vi "InstrumentSelection.vi"(8 "error in (no error)":errorcluster, 9 "Verify GPIB address":bool, 10 "Instrument type":enum16{"Supply", "LCR", "Multimeter"}(ring), 11 "Instrument name IN":string(combo)) -> (0 "error out":errorcluster, 1 "Instrument name OUT":string, 2 "LCR":refnum<class "LCRControl.lvclass">, 3 "Supply":refnum<class "SupplyControl.lvclass">, 5 "Multimeter":refnum<class "MultimeterControl.lvclass">)   [LabVIEW 2018, in "InstrControl.lvclass"]
uses:
  InstrControl.lvclass
  SupplyControl/SupplyControl.lvclass
  C:/ProbeTestSoftware2019/itk-strip-sensor-qc/InstrControl/InstrControl.lvclass
  LCRControl/LCRControl.lvclass
  MultimeterControl/MultimeterControl.lvclass
  SupplyControl/Keithley 2410/KE2410.lvclass
  C:/ProbeTestSoftware2019/itk-strip-sensor-qc/InstrControl/SupplyControl/SupplyControl.lvclass
  SupplyControl/Keithley 6517/KE6517.lvclass
  SupplyControl/Keithley 487/KE487.lvclass
  SupplyControl/Keithley 2657A/KE2657A.lvclass
  SupplyControl/Keithley 236 & 237/KE236.lvclass
  LCRControl/WK6440B/WK6440B.lvclass
  C:/ProbeTestSoftware2019/itk-strip-sensor-qc/InstrControl/LCRControl/LCRControl.lvclass
  LCRControl/WK6425/WK6425.lvclass
  MultimeterControl/Keithley 2000/KE2000.lvclass
  C:/ProbeTestSoftware2019/itk-strip-sensor-qc/InstrControl/MultimeterControl/MultimeterControl.lvclass
  InstrumentSetup.vi
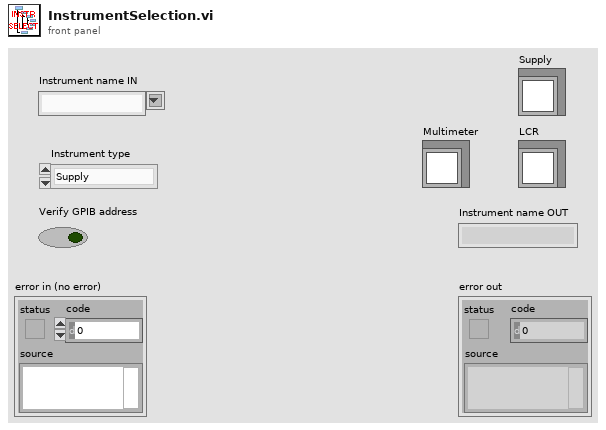
[diagram p1: front panel]
types:
  T1 = cluster{"KE 2410":cluster{"Instrument name":string, "GPIB address":string, "Instrument type":u16}, "KE 6517":cluster{"Instrument name":string, "GPIB address":string, "Instrument type":u16}, "KE 487":cluster{"Instrument name":string, "GPIB address":string, "Instrument type":u16}, "KE 2657A":cluster{"Instrument name":string, "GPIB address":string, "Instrument type":u16}, "KE 236":cluster{"Instrument name":string, "GPIB address":string, "Instrument type":u16}, "WK 6440B":cluster{"Instrument name":string, "GPIB address":string, "Instrument type":u16}, "WK 6425":cluster{"Instrument name":string, "GPIB address":string, "Instrument type":u16}, "Pickering Matrix":cluster{"Instrument name":string, "GPIB address":string, "Instrument type":u16}, "KE 2000":cluster{"Instrument name":string, "GPIB address":string, "Instrument type":u16}}
  T2 = cluster{"current \ncompliance level":dbl, "compliance/\nmeasurement range (auto:0)":u16}
  T3 = cluster{"RC Configuration":u16, "AC amplitude [V]":dbl, "AC frequency [Hz]":i32}
  T4 = cluster{"Range":u16, "Range Value":dbl, "Function":u16}
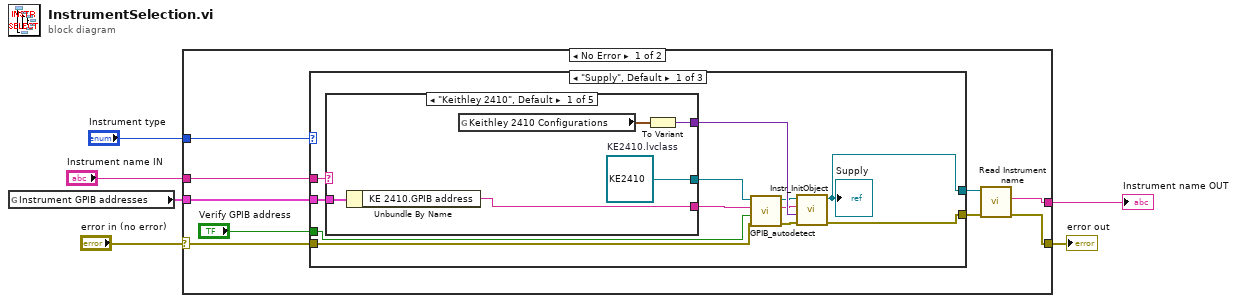
[diagram p0: block diagram]
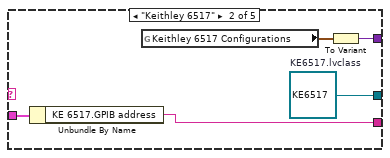
[diagram p2: hidden frame]
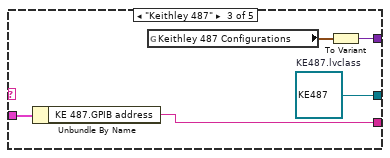
[diagram p3: hidden frame]
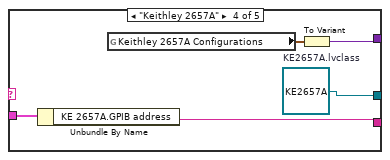
[diagram p4: hidden frame]
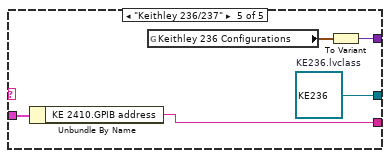
[diagram p5: hidden frame]
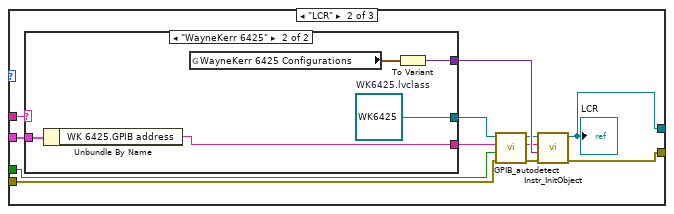
[diagram p6: hidden frame]
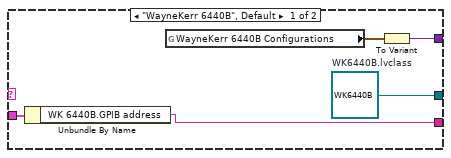
[diagram p7: hidden frame]
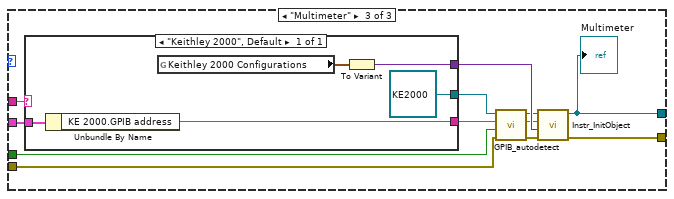
[diagram p8: hidden frame]
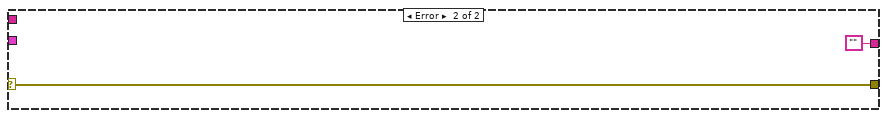
[diagram p9: hidden frame]
diagram:
  n1 = global read "InstrumentSetup.vi" "Instrument GPIB addresses"() -> (w1:T1)
  n2 = case shown="No Error" "error in (no error)" {
    selector: "error in (no error)" -> [w13 w93]
    tunnel: [w14 w93] -> w5
    tunnel: [w15 ""] -> w4
    tunnel: "Instrument type" -> [w10 _]
    tunnel: "Instrument name IN" -> [w9 _]
    tunnel: w1 -> [w8 _]
    frame No Error {
      n3 = case shown="\"Supply\", Default" w10 {
        tunnel: w9 -> [w27 w64 w86]
        tunnel: [w26 w62 w84] -> w12
        tunnel: w13 -> [w18 w59 w76]
        tunnel: [w25 w63 w85] -> w11
        tunnel: w8 -> [w24 w61 w83]
        tunnel: "Verify GPIB address" -> [w17 w53 w81]
        frame "Supply", Default {
          n4 = case shown="\"Keithley 2410\", Default" w27 {
            tunnel: [w32 w37 w42 w43 w52] -> w20
            tunnel: w24 -> [w31 w36 w41 w45 w51]
            tunnel: [w30 w35 w40 w44 w50] -> w22
            tunnel: [w28 w33 w39 w46 w48] -> w23
            frame "Keithley 2410", Default {
              w32 = refnum<class "KE2410.lvclass"> refnum  # KE2410.lvclass
              n5 = Unbundle By Name(w31) -> ("KE 2410.GPIB address"=w30:string)
              n6 = global read "InstrumentSetup.vi" "Keithley 2410 Configurations"() -> (w29:cluster{"Current Limit":sgl})
              n7 = To Variant(anything=w29) -> (Variant=w28:variant)
            }
            frame "Keithley 6517" {
              w37 = refnum<class "KE6517.lvclass"> refnum  # KE6517.lvclass
              n8 = Unbundle By Name(w36) -> ("KE 6517.GPIB address"=w35:string)
              n9 = global read "InstrumentSetup.vi" "Keithley 6517 Configurations"() -> (w34:cluster{"Current Limit":u16})
              n10 = To Variant(anything=w34) -> (Variant=w33:variant)
            }
            frame "Keithley 487" {
              w42 = refnum<class "KE487.lvclass"> refnum  # KE487.lvclass
              n11 = Unbundle By Name(w41) -> ("KE 487.GPIB address"=w40:string)
              n12 = global read "InstrumentSetup.vi" "Keithley 487 Configurations"() -> (w38:cluster{"Compliance":u16, "Range:":u16})
              n13 = To Variant(anything=w38) -> (Variant=w39:variant)
            }
            frame "Keithley 2657A" {
              w43 = refnum<class "KE2657A.lvclass"> refnum  # KE2657A.lvclass
              n14 = Unbundle By Name(w45) -> ("KE 2657A.GPIB address"=w44:string)
              n15 = global read "InstrumentSetup.vi" "Keithley 2657A Configurations"() -> (w47:cluster{"Current Limit":sgl})
              n16 = To Variant(anything=w47) -> (Variant=w46:variant)
            }
            frame "Keithley 236/237" {
              w52 = refnum<class "KE236.lvclass"> refnum  # KE236.lvclass
              n17 = Unbundle By Name(w51) -> ("KE 2410.GPIB address"=w50:string)
              n18 = global read "InstrumentSetup.vi" "Keithley 236 Configurations"() -> (w49:T2)
              n19 = To Variant(anything=w49) -> (Variant=w48:variant)
            }
          }
          n20 = call-dynamic "GPIB_autodetect.vi"("error in (no error)"=w18, "Verify GPIB address"=w17, "Instrument GPIB address in"=w22, "InstrControl in"=w20) -> ("error out"=w16:errorcluster, "Instrument GPIB address"=w21:string, "InstrControl out"=w19:refnum<class "SupplyControl.lvclass">)  [unwired: 5 in]
          n21 = call-dynamic "Instr_InitObject.vi"("error in (no error)"=w16, "Instrument Configuration"=w23, "GPIB address"=w21, "SupplyControl in"=w19) -> ("error out"=w25:errorcluster, "SupplyControl out"=w26:refnum<class "SupplyControl.lvclass">)  [unwired: 6 in]
          "Supply" <- w26
        }
        frame "LCR" {
          n22 = case shown="\"WayneKerr 6425\"" w64 {
            tunnel: [w69 w74] -> w55
            tunnel: w61 -> [w68 w73]
            tunnel: [w67 w72] -> w57
            tunnel: [w66 w71] -> w60
            frame "WayneKerr 6440B", Default {
              w69 = refnum<class "WK6440B.lvclass"> refnum  # WK6440B.lvclass
              n23 = Unbundle By Name(w68) -> ("WK 6440B.GPIB address"=w67:string)
              n24 = global read "InstrumentSetup.vi" "WayneKerr 6440B Configurations"() -> (w65:T3)
              n25 = To Variant(anything=w65) -> (Variant=w66:variant)
            }
            frame "WayneKerr 6425" {
              w74 = refnum<class "WK6425.lvclass"> refnum  # WK6425.lvclass
              n26 = Unbundle By Name(w73) -> ("WK 6425.GPIB address"=w72:string)
              n27 = global read "InstrumentSetup.vi" "WayneKerr 6425 Configurations"() -> (w70:T3)
              n28 = To Variant(anything=w70) -> (Variant=w71:variant)
            }
          }
          n29 = call-dynamic "GPIB_autodetect.vi"("error in (no error)"=w59, "Verify GPIB address"=w53, "Instrument GPIB address in"=w57, "InstrControl in"=w55) -> ("error out"=w58:errorcluster, "Instrument GPIB address"=w56:string, "InstrControl out"=w54:refnum<class "LCRControl.lvclass">)  [unwired: 5 in]
          n30 = call-dynamic "Instr_InitObject.vi"("error in (no error)"=w58, "Instrument Configuration"=w60, "GPIB Address"=w56, "LCRControl in"=w54) -> ("error out"=w63:errorcluster, "LCRControl out"=w62:refnum<class "LCRControl.lvclass">)  [unwired: 6 in]
          "LCR" <- w62
        }
        frame "Multimeter" {
          n31 = case shown="\"Keithley 2000\", Default" w86 {
            tunnel: [refnum<class "KE2000.lvclass"> refnum ("KE2000.lvclass")] -> w77
            tunnel: w83 -> [w90]
            tunnel: [w89] -> w80
            tunnel: [w88] -> w82
            frame "Keithley 2000", Default {
              n32 = Unbundle By Name(w90) -> ("KE 2000.GPIB address"=w89:string)
              n33 = global read "InstrumentSetup.vi" "Keithley 2000 Configurations"() -> (w87:T4)
              n34 = To Variant(anything=w87) -> (Variant=w88:variant)
            }
          }
          n35 = call-dynamic "GPIB_autodetect.vi"("error in (no error)"=w76, "Verify GPIB address"=w81, "Instrument GPIB address in"=w80, "InstrControl in"=w77) -> ("error out"=w75:errorcluster, "Instrument GPIB address"=w79:string, "InstrControl out"=w78:refnum<class "KE2000.lvclass">)  [unwired: 5 in]
          n36 = call-dynamic "Instr_InitObject.vi"("error in (no error)"=w75, "Instrument Configuration"=w82, "GPIB Address"=w79, "KE2000 in"=w78) -> ("error out"=w85:errorcluster, "KE2000 out"=w84:refnum<class "KE2000.lvclass">)  [unwired: 6 in]
          "Multimeter" <- w84
        }
      }
      n37 = call-dynamic "Read Instrument name.vi"("error in (no error)"=w11, "InstControl in"=w12) -> ("error out"=w14:errorcluster, "Instrument name"=w15:string)  [unwired: 7 in, 1 out]
    }
    frame Error {
    }
  }
  "error out" <- w5
  "Instrument name OUT" <- w4
